vi "fgv_Gslam_edge.vi"(7 "cmd":T1, 11 "pf-val":T3={"e"=[[0.04000000000000001]], "omega"=[[0.04000000000000001]], "d1"=0.0, "d2"=0.0, "yaw1"=0.0, "yaw2"=0.0, "angle1"=0.0, "angle2"=0.0, "id1"=0, "id2"=0}) -> (3 "pf-val out":T3={"e"=[[0.04000000000000001]], "omega"=[[0.04000000000000001]], "d1"=0.0, "d2"=0.0, "yaw1"=0.0, "yaw2"=0.0, "angle1"=0.0, "angle2"=0.0, "id1"=0, "id2"=0})   [LabVIEW 2019]
uses:
  <vilib>/Analysis/Matrix/Datatypes/RealMatrix.ctl
  Ctrl/cmd_ini-RW.ctl
  <vilib>/Analysis/Matrix/NI_Matrix.lvlib
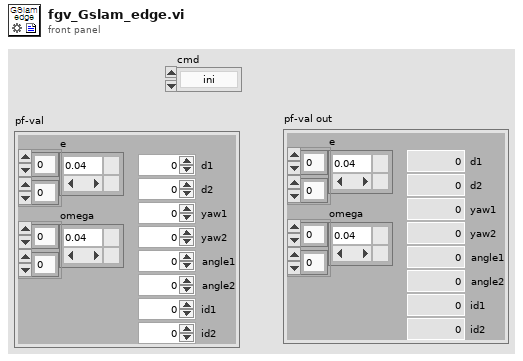
[diagram p1: front panel]
types:
  T1 = typedef "cmd_ini-RW.ctl" = enum16{"ini", "read", "write"}
  T2 = typedef "NI_Matrix.lvlib/RealMatrix.ctl" = dbl[][]
  T3 = cluster{"e":T2, "omega":T2, "d1":dbl, "d2":dbl, "yaw1":dbl, "yaw2":dbl, "angle1":dbl, "angle2":dbl, "id1":u32, "id2":u32}
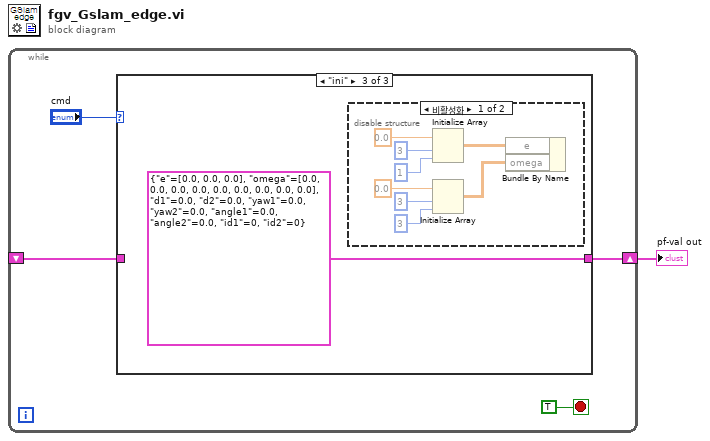
[diagram p0: block diagram]
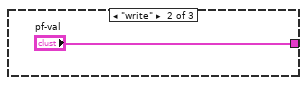
[diagram p3: hidden frame]
diagram:
  n1 = while {
    shift-right: [w4] -> w1
    shift-left: _ -> [w3]
    stop <- TRUE stop-if-true
    n2 = case shown="\"ini\"" "cmd" {
      tunnel: [w6 "pf-val" T3 {"e"=[[0.0], [0.0], [0.0]], "omega"=[[0.0, 0.0, 0.0], [0.0, 0.0, 0.0], [0.0, 0.0, 0.0]], "d1"=0.0, "d2"=0.0, "yaw1"=0.0, "yaw2"=0.0, "angle1"=0.0, "angle2"=0.0, "id1"=0, "id2"=0} ("pf-val")] -> w4
      tunnel: w3 -> [w6 _ _]
      frame "read", Default {
      }
      frame "write" {
      }
      frame "ini" {
        n3 = disable-structure shown="비활성화" {
          frame Disabled {
            n4 = Initialize Array(0.0 ("원소"), 3 ("차원 크기"), 1 ("차원 크기")) -> (w10:dbl[][])
            n5 = Initialize Array(0.0 ("원소"), 3 ("차원 크기"), 3 ("차원 크기")) -> (w9:dbl[][])
            n6 = Bundle By Name("e"=w10, "omega"=w9) -> ()  [unwired: 1 in, 1 out]
          }
          frame Enabled {
          }
        }
      }
    }
  }
  "pf-val out" <- w1
